vi "Pass If.vi"(7 "Description":string, 8 "error in (no error)":errorcluster, 9 "Message":string, 10 "Pass?":bool, 11 "LUnit Test Case In":refnum<class "LUnit Test Case.lvclass">) -> (0 "error out":errorcluster, 3 "LUnit Test Case Out":refnum<class "LUnit Test Case.lvclass">)   [LabVIEW 2020, in "LUnit Test Case.lvclass"]
doc: "Generates a pass result for the calling test method if the conditional input is true. A description and message may be provided."
uses:
  LUnit Test Case.lvclass
  Result Types/Assertion Result/Public/TypeDefs/Assertion Type.ctl
  LUnit Test Case.lvclass/LUnit Test Case.ctl
  Private/SubVIs/Add test result.vi
  Result Types/Case Result/Public/Record Assertion Result.vi
  Result Types/Method Result/Public/Aggregate Assertion Results.vi
  Result Types/Method Result/Private/Merge Status.vi
  Result Types/Method Result/Private/Concatenate result strings.vi
  Result Types/Assertion Result/Assertion Result.lvlib
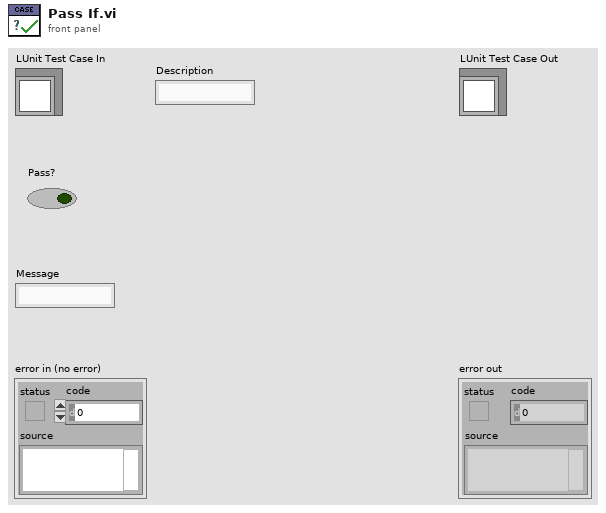
[diagram p1: front panel]
types:
  T1 = typedef "Assertion Result.lvlib/Assertion Type.ctl" = enum16{"None", "Pass", "Fail", "Skip", "Pass if Equal", "Fail if Equal", "Pass if Error", "Fail if Error", "Pass if", "Fail if"}
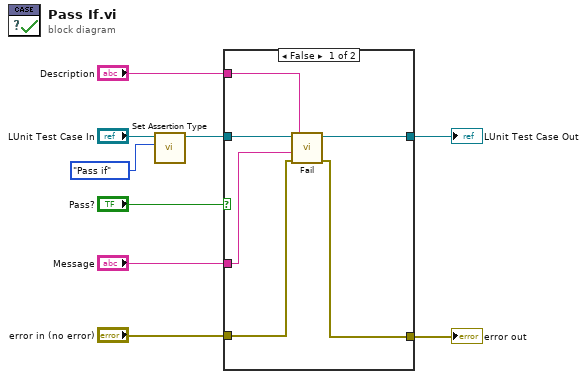
[diagram p0: block diagram]
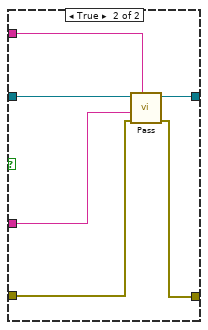
[diagram p2: hidden frame]
diagram:
  n1 = call "Set Assertion Type.vi"("Assertion Type"=Assertion_Type."Pass if", "LUnit Test Case In"="LUnit Test Case In") -> ("LUnit Test Case Out"=w3:refnum<class "LUnit Test Case.lvclass">)  [unwired: 9 in]
  n2 = case shown="False" "Pass?" {
    tunnel: [w14 w21] -> w9
    tunnel: [w13 w17] -> w8
    tunnel: "Description" -> [w11 w19]
    tunnel: "Message" -> [w12 w18]
    tunnel: w3 -> [w15 w20]
    tunnel: "error in (no error)" -> [w10 w16]
    frame False {
      n3 = call "Fail.vi"("Description"=w11, "error in (no error)"=w10, "Message"=w12, "LUnit Test Case In"=w15) -> ("error out"=w13:errorcluster, "LUnit Test Case Out"=w14:refnum<class "LUnit Test Case.lvclass">)  [unwired: 6 in]
    }
    frame True {
      n4 = call "Pass.vi"("Description"=w19, "error in (no error)"=w16, "Message"=w18, "LUnit Test Case In"=w20) -> ("error out"=w17:errorcluster, "LUnit Test Case Out"=w21:refnum<class "LUnit Test Case.lvclass">)  [unwired: 6 in]
    }
  }
  "error out" <- w8
  "LUnit Test Case Out" <- w9
